vi "Read Data.vi"(8 "ErrorIn":errorcluster, 11 "VISAIn":refnum<visa-resource-name>) -> (0 "ErrorOut":errorcluster, 2 "Read Data":string, 3 "Current Data":string)   [LabVIEW 2017, in "I28Drivers.lvlib"]
uses:
  I28Drivers.lvlib
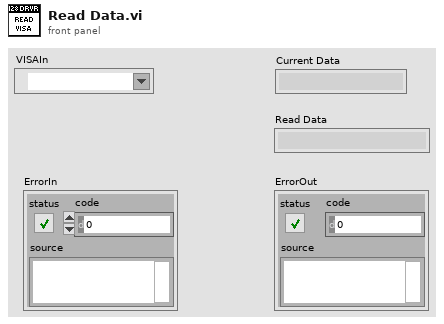
[diagram p1: front panel]
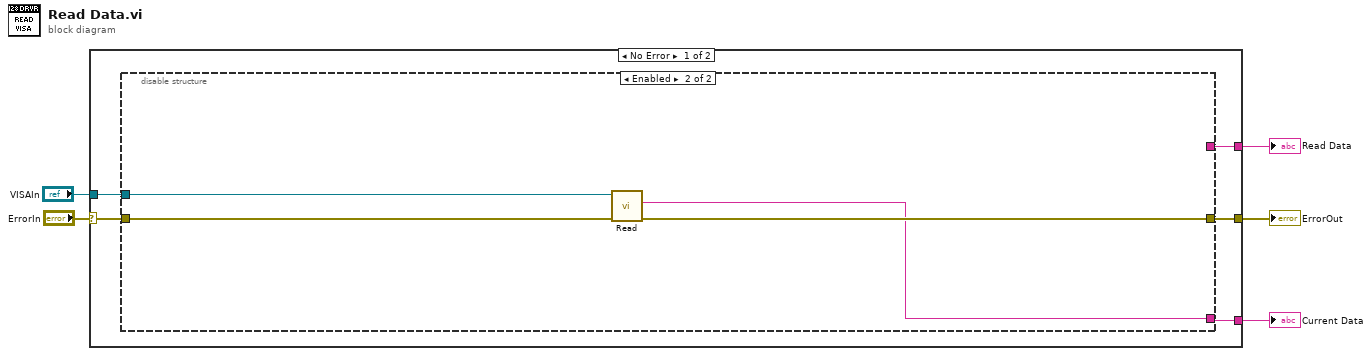
[diagram p0: block diagram]
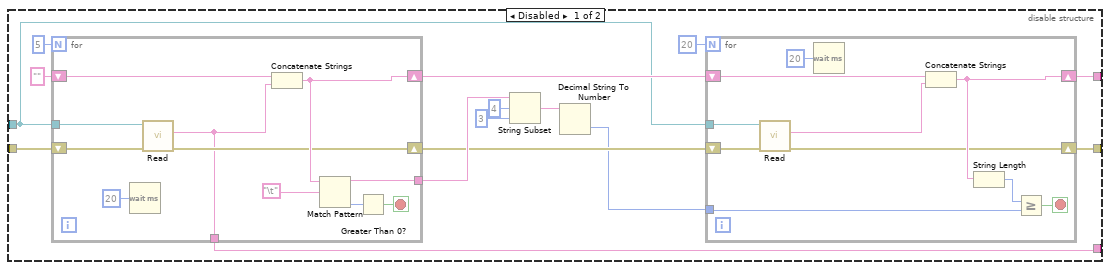
[diagram p2: hidden frame]
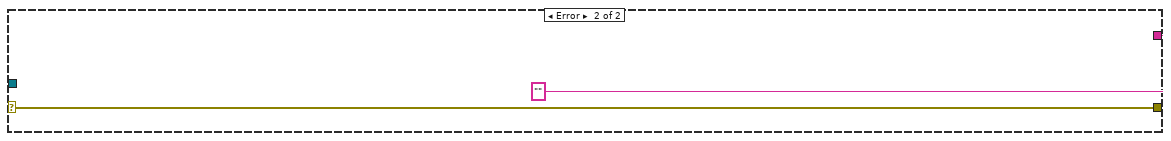
[diagram p3: hidden frame]
diagram:
  n1 = case shown="No Error" "ErrorIn" {
    selector: "ErrorIn" -> [w10 w52]
    tunnel: [w8 w52] -> w5
    tunnel: [w9 "" ("read buffer")] -> w3
    tunnel: "VISAIn" -> [w7 _]
    tunnel: [w6 _] -> w1
    frame No Error {
      n2 = disable-structure shown="Enabled" {
        disable-tunnel: w10 -> [w25 w50]
        disable-tunnel: [w14 _] -> w9
        disable-tunnel: [w13 w48] -> w8
        disable-tunnel: w7 -> [w12 w49]
        disable-tunnel: [w11 w47] -> w6
        frame Disabled {
          n3 = for {
            N: 5 -> [_]
            shift-right: [w38] -> w16
            shift-left: w25 -> [w39]
            shift-right: [w41] -> w19
            shift-left: "" ("read buffer") -> [w42]
            tunnel: [w40] -> w22
            tunnel: w12 -> [w37]
            tunnel: [w36] -> w11
            stop <- w43 stop-if-true
            n4 = Wait (ms)(milliseconds to wait=u32 20) -> ()  [unwired: 1 out]
            n5 = call "Read.vi"("ErrorIn"=w39, "VISAIn"=w37) -> ("ErrorOut"=w38:errorcluster, "Data"=w36:string)  [unwired: 7 in, 1 out]
            n6 = Concatenate Strings(w42, w36) -> (w41:string)
            n7 = Match Pattern(string=w41, regular expression="\t") -> (before substring=w40:string, offset past match=w44:i32)  [unwired: 1 in, 2 out]
            n8 = Greater Than 0?(x=w44) -> (x > 0?=w43:bool)
          }
          n9 = String Subset(string=w22, offset (0)=4, length (rest)=3 ("length (rest)")) -> (substring=w18:string)
          n10 = Decimal String To Number(string=w18) -> (number=w15:i32)  [unwired: 2 in, 1 out]
          n11 = for {
            N: 20 -> [_]
            shift-right: [w28] -> w13
            shift-left: w16 -> [w29]
            shift-right: [w33] -> w14
            shift-left: w19 -> [w34]
            tunnel: w15 -> [w30]
            tunnel: w12 -> [w26]
            stop <- w32 stop-if-true
            n12 = call "Read.vi"("ErrorIn"=w29, "VISAIn"=w26) -> ("ErrorOut"=w28:errorcluster, "Data"=w27:string)  [unwired: 7 in, 1 out]
            n13 = Wait (ms)(milliseconds to wait=u32 20) -> ()  [unwired: 1 out]
            n14 = Concatenate Strings(w34, w27) -> (w33:string)
            n15 = String Length(string=w33) -> (length=w31:i32)
            n16 = Greater Or Equal?(x=w31, y=w30) -> (x >= y?=w32:bool)
          }
        }
        frame Enabled {
          n17 = call "Read.vi"("ErrorIn"=w50, "VISAIn"=w49) -> ("ErrorOut"=w48:errorcluster, "Data"=w47:string)  [unwired: 7 in, 1 out]
        }
      }
    }
    frame Error {
    }
  }
  "Read Data" <- w3
  "ErrorOut" <- w5
  "Current Data" <- w1
